vi "Write Frequencies.vi"(8 "error in (no error)":errorcluster, 10 "Frequencies":dbl[](array[numeric]), 11 "Spectrum Analyzer in":refnum<class "Spectrum Analyzer.lvclass">) -> (0 "error out":errorcluster, 3 "Spectrum Analyzer out":refnum<class "Spectrum Analyzer.lvclass">)   [LabVIEW 2015, in "Spectrum Analyzer.lvclass"]
uses:
  Spectrum Analyzer.lvclass
  Spectrum Analyzer.lvclass/Spectrum Analyzer.ctl
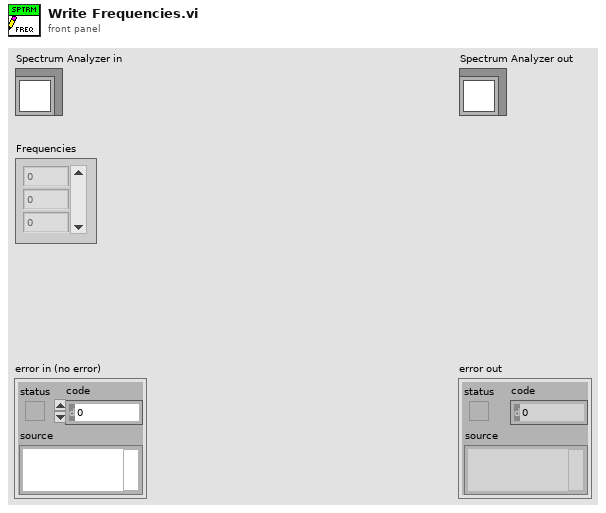
[diagram p1: front panel]
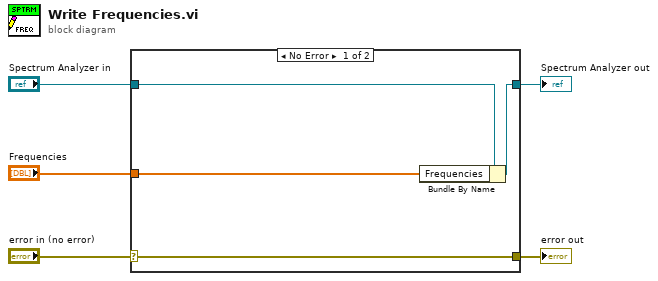
[diagram p0: block diagram]
diagram:
  n1 = case shown="No Error" "error in (no error)" {
    selector: "error in (no error)" -> [w9 w10]
    tunnel: [w9 w10] -> w4
    tunnel: [w7 w11] -> w2
    tunnel: "Spectrum Analyzer in" -> [w8 w11]
    tunnel: "Frequencies" -> [w6 _]
    frame No Error {
      n2 = Bundle By Name(cluster=w8, "Frequencies"=w6) -> (w7:refnum<class "Spectrum Analyzer.lvclass">)
    }
    frame Error {
    }
  }
  "error out" <- w4
  "Spectrum Analyzer out" <- w2
